vi "GetCtrlListGen.vi"(8 "ErrorIn(No Error)":errorcluster caption="entrée d'erreur (pas d'erreur)", 11 "CommandRef":path) -> (0 "sortie d'erreur":errorcluster, 2 "ControlsRefs":refnum<vi>[](array[refnum]), 3 "ControlsNames":string[](array[string]))   [LabVIEW 2019]
panel:
  in  "InclTabCTrl":bool
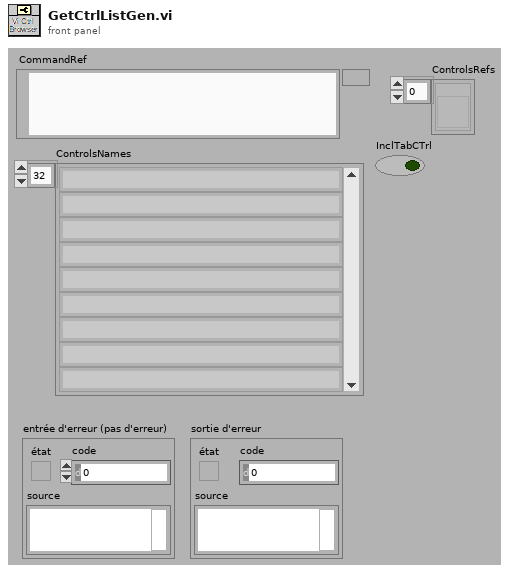
[diagram p1: front panel]
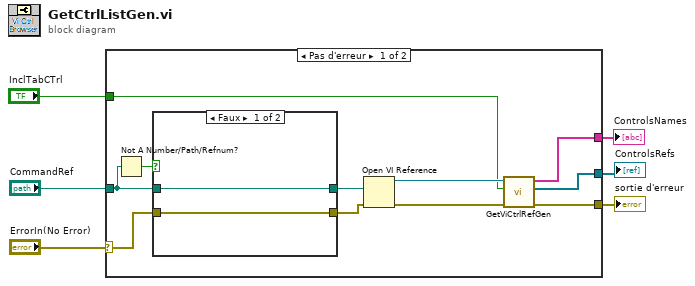
[diagram p0: block diagram]
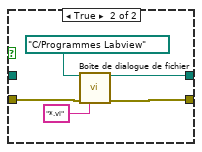
[diagram p2: hidden frame]
diagram:
  n1 = case shown="Pas d'erreur" "ErrorIn(No Error)" {
    selector: "ErrorIn(No Error)" -> [w13 w25]
    tunnel: [w9 w25] -> w5
    tunnel: "CommandRef" -> [w15 _]
    tunnel: [w8 _] -> w3
    tunnel: [w10 _] -> w2
    tunnel: "InclTabCTrl" -> [w7 _]
    frame No Error {
      n2 = Not A Number/Path/Refnum?(number/path/refnum=w15) -> (NaN/Path/Refnum?=w17:bool)
      n3 = case shown="Faux" w17 {
        tunnel: [w19 w22] -> w16
        tunnel: w15 -> [w19 _]
        tunnel: [w18 w21] -> w14
        tunnel: w13 -> [w18 w20]
        frame False {
        }
        frame True {
          n4 = call "Boîte de dialogue de fichier"("start path"=path "C:/Programmes Labview", "error in"=w20, "pattern (all files)"="*.vi") -> ("selected path"=w22:path, "error out"=w21:errorcluster)  [unwired: 9 in, 2 out]
        }
      }
      n5 = Open VI Reference(vi path=w16, error in (no error)=w14) -> (vi reference=w12:refnum<vi>, error out=w11:errorcluster)  [unwired: 4 in]
      n6 = call <userlib>:"GetViCtrlRefGen.vi"("ErrorIn(No Error)"=w11, "InclTabCTrl"=w7, "VIRef"=w12) -> ("sortie d'erreur"=w9:errorcluster, "ControlsRefs"=w8:refnum<vi>[], "ControlsNames"=w10:string[])  [unwired: 6 in]
    }
    frame Error {
    }
  }
  "sortie d'erreur" <- w5
  "ControlsRefs" <- w3
  "ControlsNames" <- w2
